vi "PerformCodeExchange.vi"(4 "client secret":string, 6 "client id":string, 7 "token request uri":string="https://api.netatmo.com/oauth2/token ", 8 "error in (no error)":errorcluster, 9 "redirect uri":string, 11 "code":string) -> (0 "error out":errorcluster, 3 "token response (JSON)":string)   [LabVIEW 2020, in "Netatmo-WeatherStation.lvlib"]
uses:
  <vilib>/httpClient/POSTBuffer.vi
  Netatmo-WeatherStation.lvlib
  <vilib>/httpClient/LabVIEWHTTPClient.lvlib
  <vilib>/wsapi/NI_WebServices.lvlib
panel:
  in  "grant_type":string="authorization_code"
  in  "scope":string="read_station"
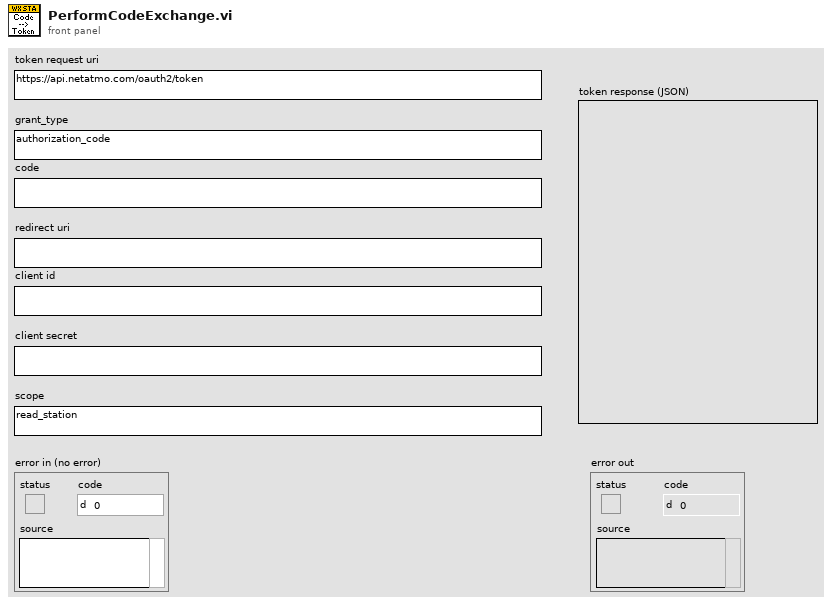
[diagram p1: front panel]
types:
  T1 = typedef "LabVIEWHTTPClient.lvlib/ClientHandle.ctl" = refnum<k1>
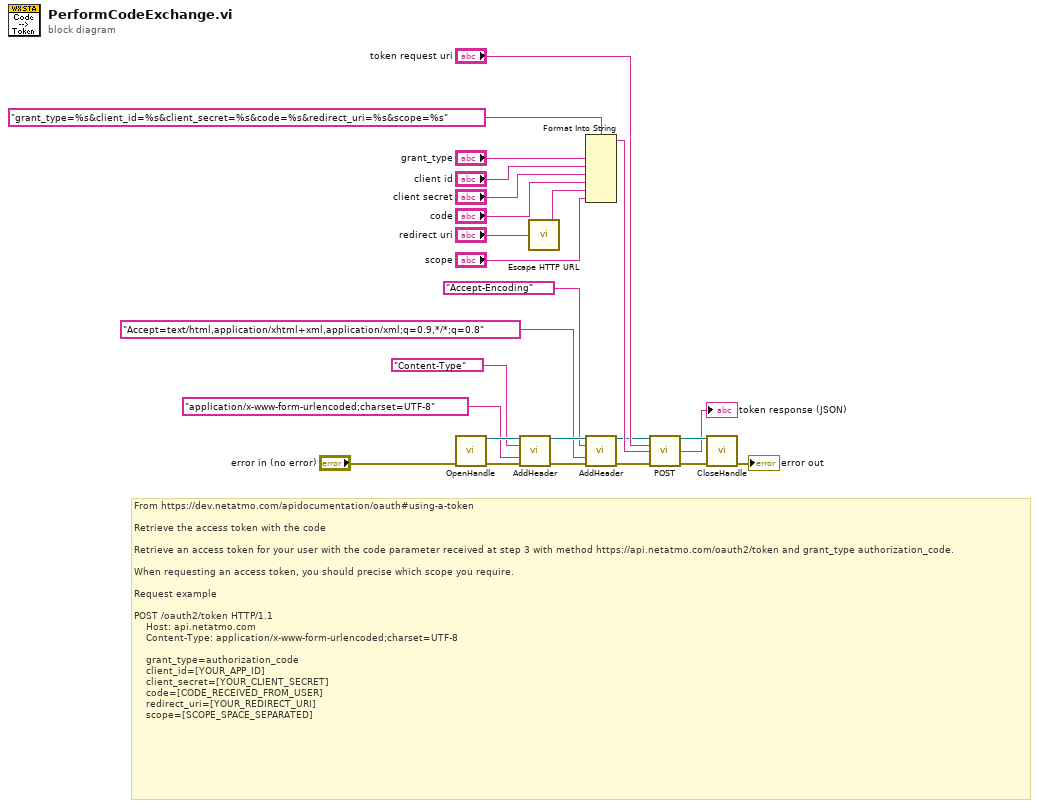
[diagram p0: block diagram]
diagram:
  # "From https://dev.netatmo.com/apidocumentation/oauth#using-a-token\n\nRetrieve the access token with the code\n\nRetrieve an access token for your user with the code parameter received at step 3 with method https://api.netatmo.com/oauth2/token and grant_type authorization_code.\n\nWhen requesting an access token, you should precise which scope you require.\n\nRequest example\n\nPOST /oauth2/token HTTP/1.1\n    Host: api.netatmo.com\n    Content-Type: application/x-www-form-urlencoded;charset=UTF-8\n\n    grant_type=authorization_code\n    client_id=[YOUR_APP_ID]\n    client_secret=[YOUR_CLIENT_SECRET]\n    code=[CODE_RECEIVED_FROM_USER]\n    redirect_uri=[YOUR_REDIRECT_URI]\n    scope=[SCOPE_SPACE_SEPARATED]"
  n1 = call <vilib>:"OpenHandle.vi"("error in (no error)"="error in (no error)") -> ("client handle out"=w24:T1, "error out"=w18:errorcluster)  [unwired: 13 in]
  n2 = call <vilib>:"AddHeader.vi"("client handle"=w24, "header"="Content-Type", "value"="application/x-www-form-urlencoded;charset=UTF-8", "error in (no error)"=w18) -> ("client handle out"=w21:T1, "error out"=w17:errorcluster)  [unwired: 10 in]
  n3 = call <vilib>:"Escape HTTP URL.vi"("unescaped string in"="redirect uri") -> ("escaped string out"=w4:string)
  n4 = Format Into String(format string="grant_type=%s&client_id=%s&client_secret=%s&code=%s&redirect_uri=%s&scope=%s", "grant_type", "client id", "client secret", "code", w4, "scope") -> (resulting string=w15:string)  [unwired: 2 in, 1 out]
  n5 = call <vilib>:"AddHeader.vi"("client handle"=w21, "header"="Accept-Encoding", "value"="Accept=text/html,application/xhtml+xml,application/xml;q=0.9,*/*;q=0.8", "error in (no error)"=w17) -> ("client handle out"=w14:T1, "error out"=w12:errorcluster)  [unwired: 10 in]
  n6 = call-poly <vilib>:"POST.vi"("client handle"=w14, "url"="token request uri", "buffer"=w15, "error in (no error)"=w12) -> ("client handle out"=w11:T1, "body"=→"token response (JSON)":string, "error out"=w10:errorcluster)  [unwired: 8 in, 1 out]
  n7 = call <vilib>:"CloseHandle.vi"("client handle"=w11, "error in (no error)"=w10) -> ("error out"=→"error out":errorcluster)  [unwired: 13 in]
